vi "LTVUnicycleCtrl_Pack_Model_Params.vi"(6 "Max Linear Vel M/S":dbl=9.0, 7 "Max X Pos Meas Tol M":dbl=0.0625, 8 "Max angular ctrl effort Rad/S":dbl=2.0, 9 "Max linear ctrl effort M/S":dbl=1.0, 10 "Max Heading Meas Tol Rad":dbl=0.2, 11 "Max Y Pos Meas Tol M":dbl=0.125) -> (3 "LTV_Unicycle_Ctrl_Model _Params":T1 {"Max Linear Vel M/S" format="%#_13g"; "Max Y Pos Meas Tol M" format="%#_13g"; "Max X Pos Meas Tol M" format="%#_13g"; "Max Heading Meas Tol Rad" format="%#_13g"; "Max angular ctrl effort Rad/S" format="%#_13g"; "Max linear ctrl effort M/S" format="%#_13g"})   [LabVIEW 2019, in "Trajectory_Library.lvlib"]
uses:
  Trajectory_Library.lvlib
  TypeDef/LTV_UNICYCLE_CONTROLLER_MODEL_PARAMS.CTL
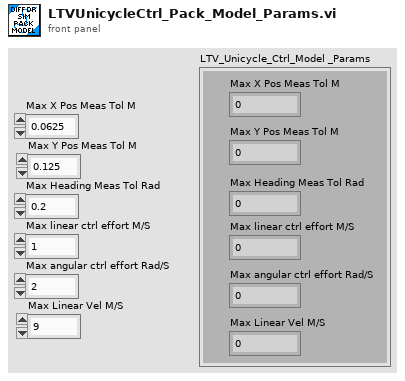
[diagram p1: front panel]
types:
  T1 = typedef "LTV_UNICYCLE_CONTROLLER_MODEL_PARAMS.CTL" = cluster{"Max linear ctrl effort M/S":dbl, "Max angular ctrl effort Rad/S":dbl, "Max Heading Meas Tol Rad":dbl, "Max X Pos Meas Tol M":dbl, "Max Y Pos Meas Tol M":dbl, "Max Linear Vel M/S":dbl}
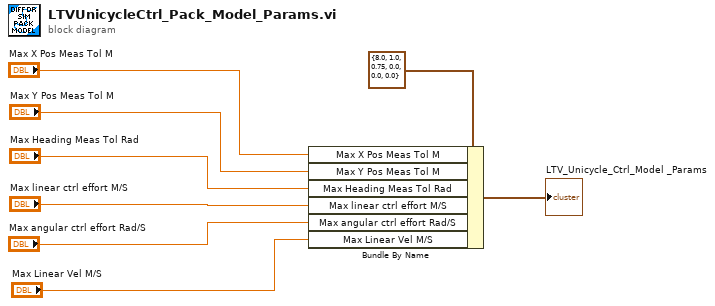
[diagram p0: block diagram]
diagram:
  n1 = Bundle By Name(cluster=T1 {"Max linear ctrl effort M/S"=8.0, "Max angular ctrl effort Rad/S"=1.0, "Max Heading Meas Tol Rad"=0.75, "Max X Pos Meas Tol M"=0.0, "Max Y Pos Meas Tol M"=0.0, "Max Linear Vel M/S"=0.0} ("SngJntArmSim_Simulation _Params"), "Max X Pos Meas Tol M"="Max X Pos Meas Tol M", "Max Y Pos Meas Tol M"="Max Y Pos Meas Tol M", "Max Heading Meas Tol Rad"="Max Heading Meas Tol Rad", "Max linear ctrl effort M/S"="Max linear ctrl effort M/S", "Max angular ctrl effort Rad/S"="Max angular ctrl effort Rad/S", "Max Linear Vel M/S"="Max Linear Vel M/S") -> (→"LTV_Unicycle_Ctrl_Model _Params":T1)
